vi "sr830_init.vi"(4 "error in (no error)":errorcluster, 6 "Sensitivity (-1: Auto gain)":i16(ring)=20 items=["Auto Gain"=-1, "2 nV/fA"=0, "5 nV/fA"=1, "10 nV/fA"=2, "20 nV/fA"=3, "50 nV/fA"=4, "100 nV/fA"=5, "200 nV/fA"=6, "500 nV/fA"=7, "1 uV/pA"=8, "2 uV/pA"=9, "5 uV/pA"=10, "10 uV/pA"=11, "20 uV/pA"=12, "50 uV/pA"=13, "100 uV/pA"=14, "200 uV/pA"=15, "500 uV/pA"=16, "1 mV/nA"=17, "2 mV/nA"=18, "5 mV/nA"=19, "10 mV/nA"=20, "20 mV/nA"=21, "50 mV/nA"=22, "100 mV/nA"=23, "200 mV/nA"=24, "500 mV/mA"=25, "1 V/uA"=26], 7 "VISA resource name":refnum<visa-resource-name>) -> (0 "error out":errorcluster, 3 "SR830":refnum<visa-resource-name>)   [LabVIEW 2016]
uses:
  <instrlib>/Stanford Research 830/Stanford Research 830.lvlib
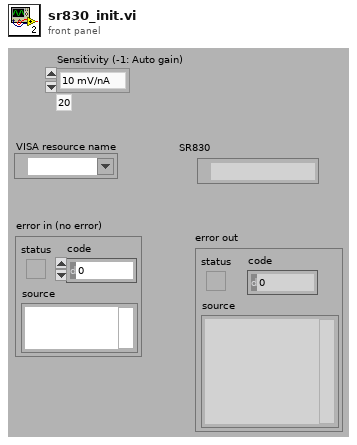
[diagram p1: front panel]
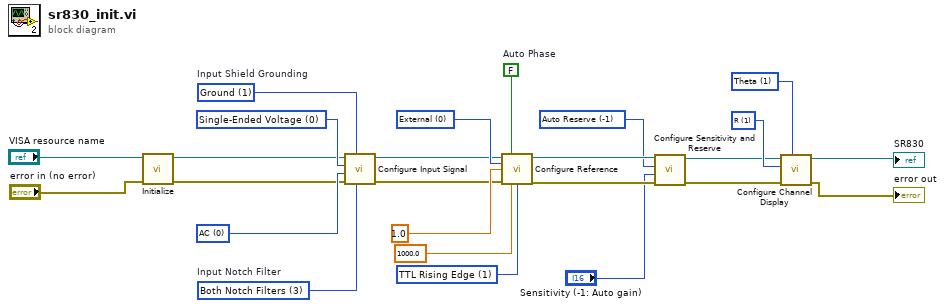
[diagram p0: block diagram]
diagram:
  w5 = u16 1 items=["Y", "Theta", "Y Noise", "Aux In 3", "Aux In 4"] ("Channel 2 Display  (0: Y)")
  w6 = u16 1 items=["X", "R", "X Noise", "Aux In 1", "Aux In 2"] ("Channel 1 Display (0: X)")
  w7 = u16 1 items=["Sine Zero Crossing", "TTL Rising Edge", "TTL Falling Edge"] ("External Reference Trigger (0: Sine Zero Crossing)")
  w8 = i16 -1 items=["Auto Reserve"=-1, "High Reserve"=0, "Normal"=1, "Low Noise"=2] ("Dynamic Reserve (-1: Auto Reserve)")
  w17 = u16 0 items=["AC", "DC"] ("Input Coupling (0: AC)")
  w16 = u16 0 items=["Single-Ended Voltage", "Differential Voltage", "1 MOhm Current Gain", "100 MOhm Current Gain"] ("Input Connection (0: Single-Ended Voltage)")
  w23 = u16 0 items=["External", "Internal"] ("Reference Source (1: Internal)")
  w20 = FALSE  # Auto Phase
  w19 = u16 3 items=["None", "Line Notch", "2x Line Notch", "Both Notch Filters"]  # Input Notch Filter
  w18 = u16 1 items=["Float", "Ground"]  # Input Shield Grounding
  n1 = call <instrlib>:"Initialize.vi"("error in (no error)"="error in (no error)", "VISA resource name"="VISA resource name") -> ("error out"=w10:errorcluster, "VISA resource name out"=w11:refnum<visa-resource-name>)  [unwired: 8 in]
  n2 = call <instrlib>:"Configure Input Signal.vi"("Input Notch Filter (0: None)"=w19, "Input Shield Grounding (0: Float)"=w18, "error in (no error)"=w10, "Input Coupling (0: AC)"=w17, "Input Connection (0: Single-Ended Voltage)"=w16, "VISA resource name"=w11) -> ("error out"=w15:errorcluster, "VISA resource name out"=w14:refnum<visa-resource-name>)  [unwired: 4 in]
  n3 = call <instrlib>:"Configure Reference.vi"("VISA resource name"=w14, "Auto Phase (T: Enabled)"=w20, "Reference Source (1: Internal)"=w23, "Sine Output Amplitude (1 V)"=1.0, "error in (no error)"=w15, "Internal Reference Frequency (1000 Hz)"=1000.0, "External Reference Trigger (0: Sine Zero Crossing)"=w7) -> ("VISA resource name out"=w21:refnum<visa-resource-name>, "error out"=w22:errorcluster)  [unwired: 7 in]
  n4 = call <instrlib>:"Configure Sensitivity and Reserve.vi"("error in (no error)"=w22, "Sensitivity (-1: Auto gain)"="Sensitivity (-1: Auto gain)", "Dynamic Reserve (-1: Auto Reserve)"=w8, "VISA resource name"=w21) -> ("error out"=w1:errorcluster, "VISA resource name out"=w2:refnum<visa-resource-name>)  [unwired: 6 in]
  n5 = call <instrlib>:"Configure Channel Display.vi"("Channel 2 Display  (0: Y)"=w5, "error in (no error)"=w1, "Channel 1 Display (0: X)"=w6, "VISA resource name"=w2) -> ("error out"=→"error out":errorcluster, "VISA resource name out"=→"SR830":refnum<visa-resource-name>)  [unwired: 6 in]
